vi "DHE_GetTimingInfo.vi"(11 "Database RefNum out":T1) -> (0 "exposure_overhead":dbl, 1 "seqs_overhead":dbl, 2 "Timing":T2 {"DET_READ_TIME" format="%.2f"; "known_overhead" format="%.2f"; "ShiftRow" format="%.2f"; "SkipRow" format="%.2f"; "SkipPixel" format="%.2f"; "PixelTime" format="%.2f"})   [LabVIEW 2016]
uses:
  Common/public/vis/CMN_TimingInfo.ctl
  DBSHAND/private/vis/DatabaseHand_RefNum.ctl
  private/vis/DHE_GBLDriverVariables.vi
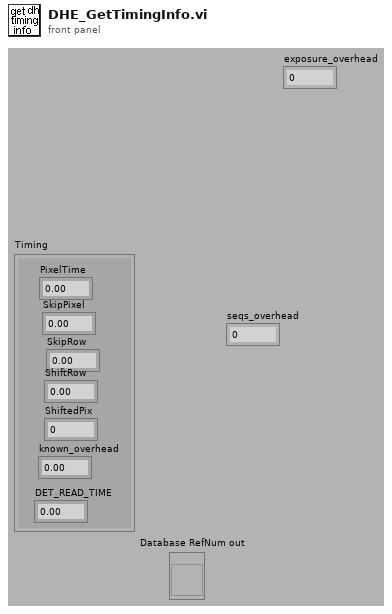
[diagram p1: front panel]
types:
  T1 = typedef "DatabaseHand_RefNum.ctl" = refnum<vi>
  T2 = typedef "CMN_TimingInfo.ctl" = cluster{"PixelTime":sgl, "SkipPixel":sgl, "SkipRow":sgl, "ShiftRow":sgl, "ShiftedPix":u16, "known_overhead":sgl, "DET_READ_TIME":sgl}
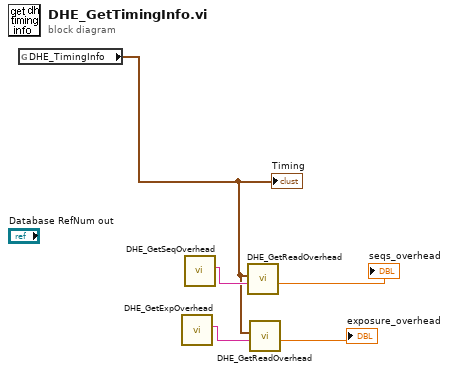
[diagram p0: block diagram]
diagram:
  n1 = global read "DHE_GBLDriverVariables.vi" "DHE_TimingInfo"() -> (w3:T2)
  "Timing" <- w3
  n2 = call "DHE_GetExpOverhead.vi"() -> ("ExpOverhead"=w2:string)  [unwired: 11 out]
  n3 = call "DHE_GetSeqOverhead.vi"() -> ("SeqOverhead"=w5:string)  [unwired: 11 out]
  n4 = call "DHE_GetReadOverhead.vi"("overhead string"=w5, "Timing"=w3) -> ("overhead"=→"seqs_overhead":dbl)  [unwired: 9 out]
  n5 = call "DHE_GetReadOverhead.vi"("overhead string"=w2, "Timing"=w3) -> ("overhead"=→"exposure_overhead":dbl)  [unwired: 9 out]
